vi "Read Legend Data.vi"(11 "Data Value Reference in":refnum<data-value>) -> (0 "error out":errorcluster, 1 "Labels[]":string[](array[string]), 2 "Legend Font":T1, 3 "Include Legend?":bool, 4 "Colors[]":u32[](array[colorbox]))   [LabVIEW 2018, in "PieChart.lvclass"]
uses:
  PieChart.lvclass
  <vilib>/Utility/miscctls.llb/LVFontTypeDef.ctl
  State Data.ctl
  <vilib>/Utility/miscctls.llb/LVBoundsTypeDef.ctl
  Pie info for Click.ctl
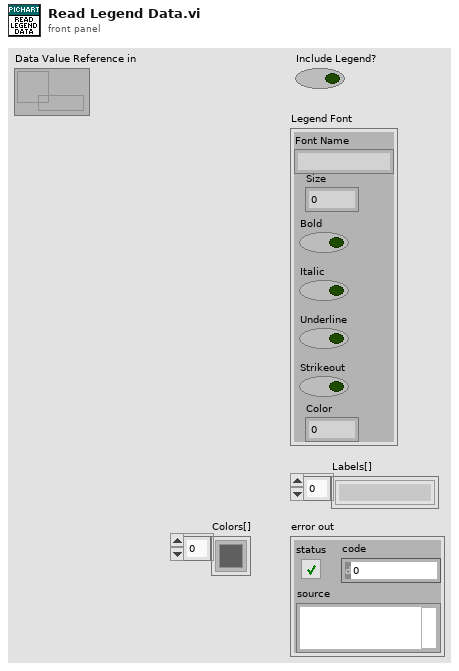
[diagram p1: front panel]
types:
  T1 = typedef "LVFontTypeDef.ctl" = cluster{"Font Name":string, "Size":u16, "Bold":bool, "Italic":bool, "Underline":bool, "Strikeout":bool, "Color":u32}
  T2 = typedef "PieChart.lvclass/State Data.ctl" = cluster{"Title":string, "Values[]":dbl[], "Labels[]":string[], "Colors[]":u32[], "Include Legend?":bool, "Include Title?":bool, "Title Font":T1, "Legend Font":T1, "Selection":i32, "Slice Positions":T3}
  T3 = typedef "PieChart.lvclass/Pie info for Click.ctl" = cluster{"Slice Positions":cluster{"Start":i16, "End":i16}[], "Center Position":T4, "Radius":i16}
  T4 = typedef "LVBoundsTypeDef.ctl" = cluster{"Width":u32, "Height":u32}
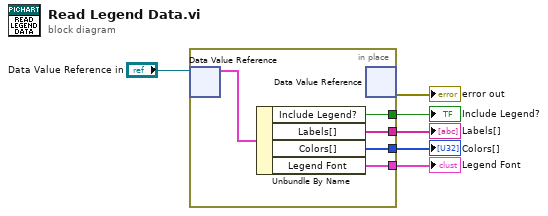
[diagram p0: block diagram]
diagram:
  n1 = in-place {
    in-place-border: [w10] -> w4
    in-place-border: [w9] -> w2
    in-place-border: [w8] -> w1
    in-place-border: [w7] -> w3
    n2 = in-place-dvr #1("Data Value Reference in") -> (w11:T2)  [unwired: 1 out]
    n3 = Unbundle By Name(w11) -> ("Include Legend?"=w10:bool, "Labels[]"=w9:string[], "Colors[]"=w8:u32[], "Legend Font"=w7:T1)
    n4 = in-place-dvr #1() -> (→"error out":errorcluster)  [unwired: 1 in, 1 out]
  }
  "Legend Font" <- w3
  "Include Legend?" <- w4
  "Labels[]" <- w2
  "Colors[]" <- w1
